vi "cover8-12.vi"(1 "H":i32=1200, 2 "W":i32=1600, 3 "Image Data":u8[](array[numeric])) -> (0 "PIC Out":u16[][](array[numeric]))   [LabVIEW 2018]
panel:
  # "将12位数据转换为8位\n输出图像数据"
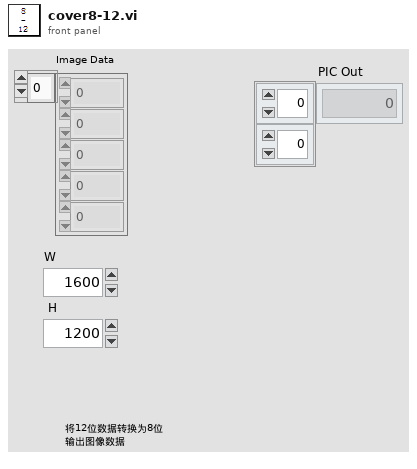
[diagram p1: front panel]
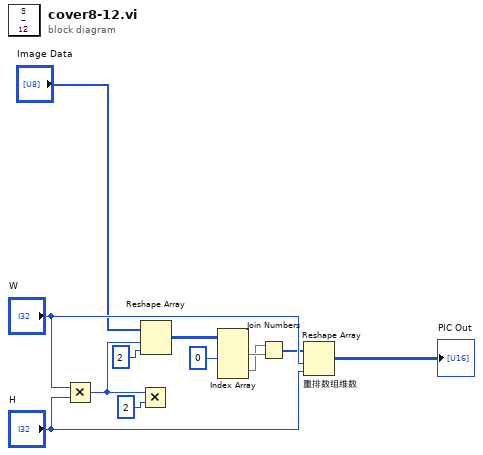
[diagram p0: block diagram]
diagram:
  n1 = Multiply(x="W", y="H") -> (x*y=w7:i32)
  n2 = Multiply(x=w7, y=2) -> ()  [unwired: 1 out]
  n3 = Reshape Array("Image Data", w7, 2 ("维数大小")) -> (w5:u8[][])
  n4 = Index Array(array=w5, index (col) #1=0 ("禁用的索引 (列)")) -> (element #1=w3:u8[], element #2=w2:u8[])  [unwired: 3 in]
  n5 = Join Numbers(hi=w2, lo=w3) -> ((hi.lo)=w1:u16[])
  n6 = Reshape Array "重排数组维数"(w1, "W", "H") -> (→"PIC Out":u16[][])
